vi "Data_folder_Path.vi"(0 "Data Type":string, 1 "FlushHierarchy":bool, 4 "Short_Name":string, 5 "seconds":dbl) -> (6 "Data Folder":path)   [LabVIEW 2015]
uses:
  Globals/Constants_global.vi
  Globals/Preference_global.vi
panel:
  out "Hierarchy":string[](array[string])
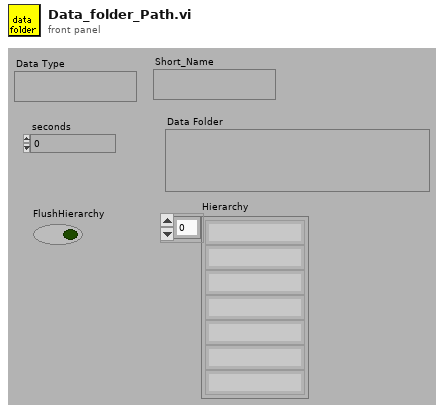
[diagram p1: front panel]
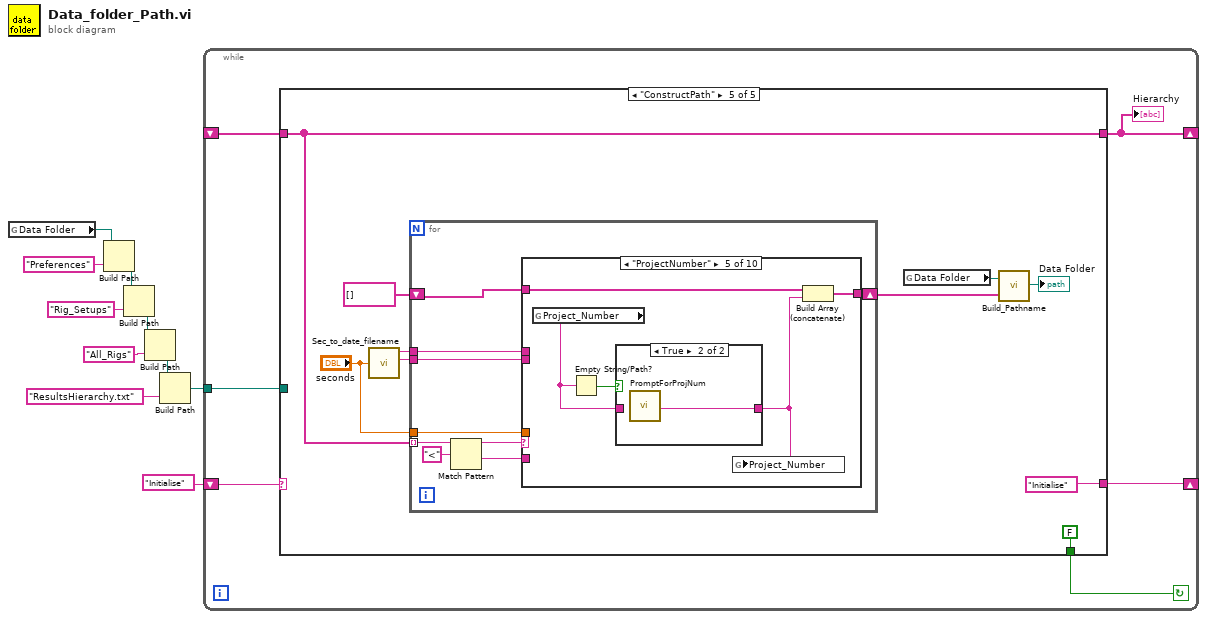
[diagram p0: block diagram]
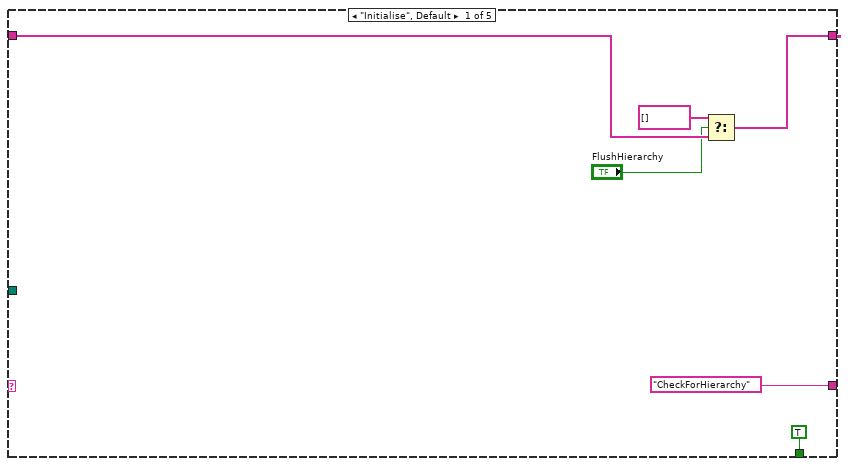
[diagram p2: hidden frame]
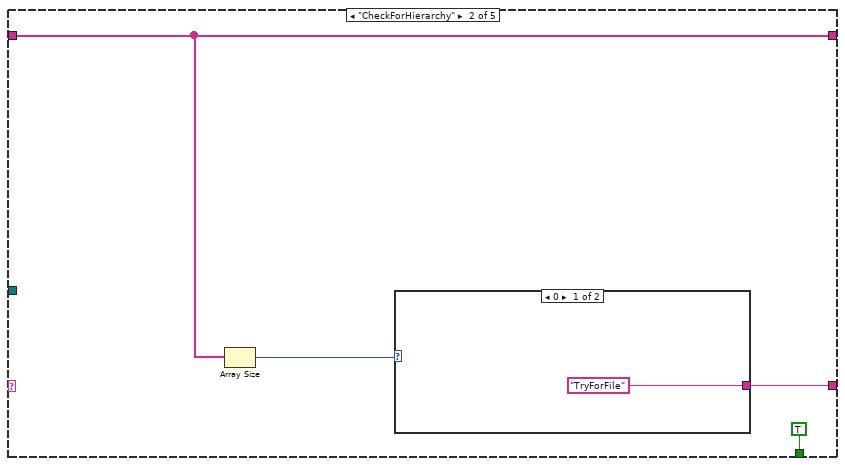
[diagram p3: hidden frame]
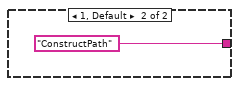
[diagram p4: hidden frame]
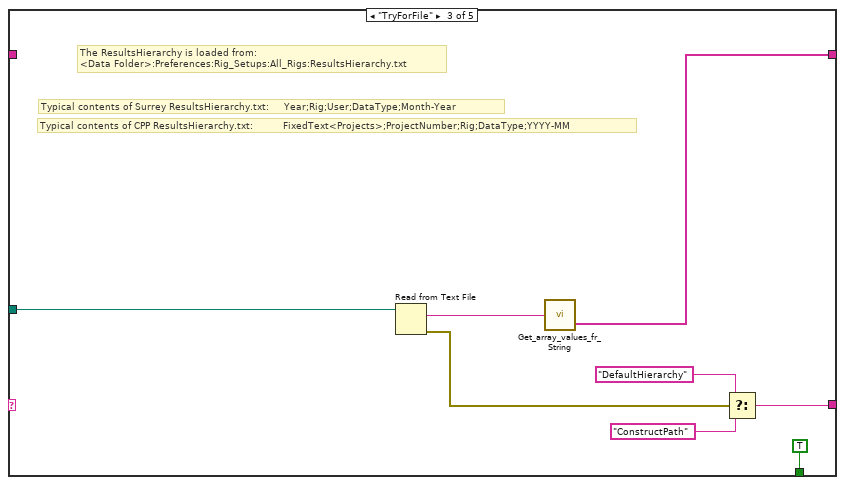
[diagram p5: hidden frame]
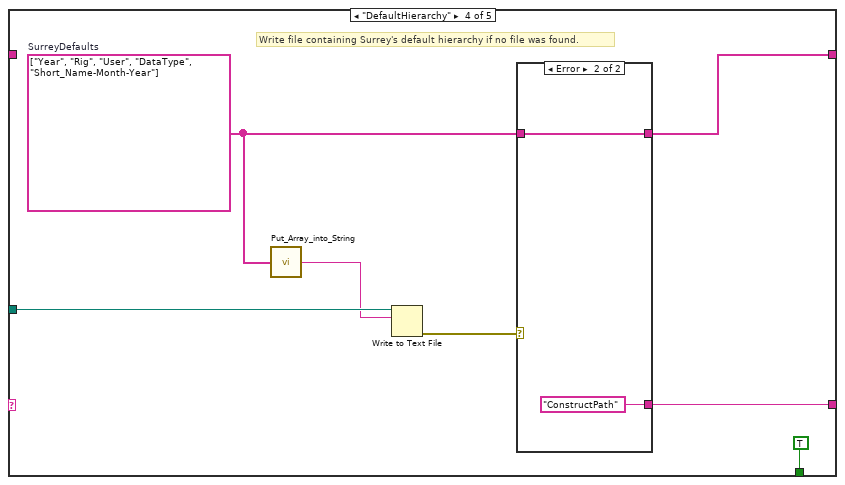
[diagram p6: hidden frame]
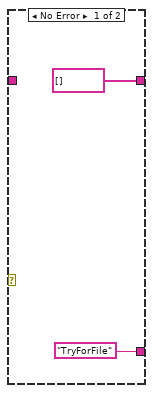
[diagram p7: hidden frame]
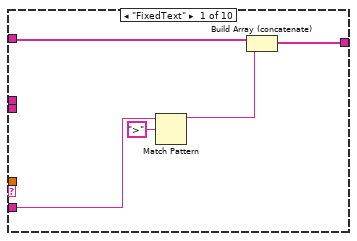
[diagram p8: hidden frame]
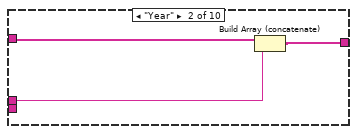
[diagram p9: hidden frame]
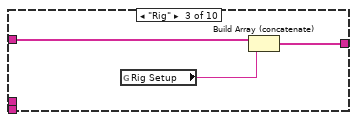
[diagram p10: hidden frame]
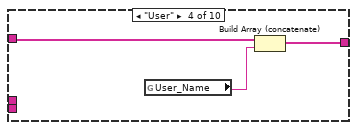
[diagram p11: hidden frame]
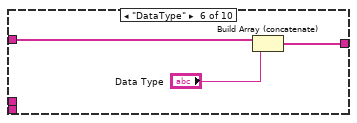
[diagram p13: hidden frame]
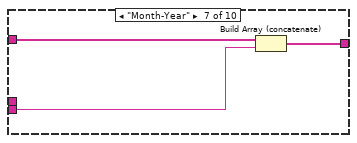
[diagram p14: hidden frame]
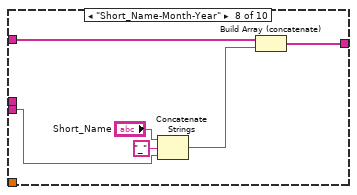
[diagram p15: hidden frame]
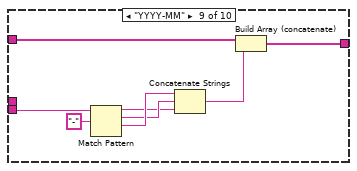
[diagram p16: hidden frame]
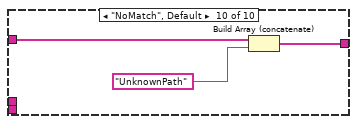
[diagram p17: hidden frame]
diagram:
  n1 = global read "Constants_global.vi" "Data Folder"() -> (w7:path)
  n2 = Build Path(base path=w7, name or relative path="Preferences") -> (appended path=w8:path)
  n3 = Build Path(base path=w8, name or relative path="Rig_Setups") -> (appended path=w1:path)
  n4 = Build Path(base path=w1, name or relative path="All_Rigs") -> (appended path=w5:path)
  n5 = Build Path(base path=w5, name or relative path="ResultsHierarchy.txt") -> (appended path=w2:path)
  n6 = while {
    shift-right: [w14] -> _
    shift-left: _ -> [w15]
    shift-right: [w13] -> _
    shift-left: "Initialise" ("t") -> [w16]
    tunnel: w2 -> [w11]
    stop <- w12 continue-if-true
    n7 = case shown="\"ConstructPath\"" w16 {
      tunnel: w15 -> [w22 w24 _ _ w50]
      tunnel: [w21 w24 w36 w39 w50] -> w14
      tunnel: ["CheckForHierarchy" ("t") w25 w35 w37 "Initialise" ("t")] -> w13
      tunnel: [TRUE TRUE TRUE TRUE FALSE] -> w12
      tunnel: w11 -> [_ _ w29 w42 _]
      frame "Initialise", Default {
        n8 = Select(t=string[] [], s="FlushHierarchy", f=w22) -> (s? t:f=w21:string[])
      }
      frame "CheckForHierarchy" {
        n9 = Array Size(array=w24) -> (size(s)=w26:i32)
        n10 = case shown="0" w26 {
          tunnel: ["TryForFile" ("t") "ConstructPath" ("t")] -> w25
          frame 0 {
          }
          frame 1, Default {
          }
        }
      }
      frame "TryForFile" {
        # "The ResultsHierarchy is loaded from:\n<Data Folder>:Preferences:Rig_Setups:All_Rigs:ResultsHierarchy.txt"
        # "Typical contents of CPP ResultsHierarchy.txt:          FixedText<Projects>;ProjectNumber;Rig;DataType;YYYY-MM"
        # "Typical contents of Surrey ResultsHierarchy.txt:     Year;Rig;User;DataType;Month-Year"
        n11 = Read from Text File(file (use dialog)=w29) -> (text=w31:string, error out=w30:errorcluster)  [unwired: 3 in, 2 out]
        n12 = call "Get_array_values_fr_String.vi"("String Value"=w31) -> ("String array"=w36:string[])  [unwired: 1 out]
        n13 = Select(t="DefaultHierarchy", s=w30, f="ConstructPath" ("t")) -> (s? t:f=w35:string)
      }
      frame "DefaultHierarchy" {
        w38 = string[] ["Year", "Rig", "User", "DataType", "Short_Name-Month-Year"]  # SurreyDefaults
        # "Write file containing Surrey's default hierarchy if no file was found."
        n14 = call "Put_Array_into_String.vi"("String array"=w38) -> ("String Value"=w41:string)
        n15 = Write to Text File(file (use dialog)=w42, text=w41) -> (error out=w40:errorcluster)  [unwired: 2 in, 2 out]
        n16 = case shown="Error" w40 {
          tunnel: [string[] [] ("SurreyDefaults") w47] -> w39
          tunnel: w38 -> [_ w47]
          tunnel: ["TryForFile" ("t") "ConstructPath" ("t")] -> w37
          frame No Error {
          }
          frame Error {
          }
        }
      }
      frame "ConstructPath" {
        n17 = call "Sec_to_date_filename.vi"("seconds"="seconds") -> ("Year"=w55:string, "Month"=w54:string)  [unwired: 2 out]
        n18 = for {
          shift-right: [w66] -> w53
          shift-left: string[] [] -> [w65]
          tunnel: w50 -> [w61] mode=indexing
          tunnel: w54 -> [w64]
          tunnel: w55 -> [w63]
          tunnel: "seconds" -> [w62]
          n19 = Match Pattern(string=w61, regular expression="<") -> (before substring=w60:string, after substring=w58:string)  [unwired: 1 in, 2 out]
          n20 = case shown="\"ProjectNumber\"" w60 {
            tunnel: [w71 w74 w76 w80 w85 w90 w93 w99 w105 w110] -> w66
            tunnel: w65 -> [w70 w73 w75 w78 w84 w89 w92 w98 w104 w109]
            tunnel: w64 -> [_ _ _ _ _ _ w91 w95 w107 _]
            tunnel: w63 -> [_ w72 _ _ _ _ _ _ _ _]
            tunnel: w62 -> [_ _ _ _ _ _ _ _ _ _]
            tunnel: w58 -> [w69 _ _ _ _ _ _ _ _ _]
            frame "FixedText" {
              n21 = Match Pattern(string=w69, regular expression=">") -> (before substring=w67:string)  [unwired: 1 in, 3 out]
              n22 = Build Array (concatenate)(w70, w67) -> (w71:string[])
            }
            frame "Year" {
              n23 = Build Array (concatenate)(w73, w72) -> (w74:string[])
            }
            frame "Rig" {
              n24 = global read "Preference_global.vi" "Rig Setup"() -> (w77:string)
              n25 = Build Array (concatenate)(w75, w77) -> (w76:string[])
            }
            frame "User" {
              n26 = global read "Preference_global.vi" "User_Name"() -> (w79:string)
              n27 = Build Array (concatenate)(w78, w79) -> (w80:string[])
            }
            frame "ProjectNumber" {
              n28 = global read "Preference_global.vi" "Project_Number"() -> (w81:string)
              n29 = Empty String/Path?(string/path=w81) -> (empty?=w83:bool)
              n30 = case shown="True" w83 {
                tunnel: [w86 w87] -> w82
                tunnel: w81 -> [w86 _]
                frame False {
                }
                frame True {
                  n31 = call "PromptForProjNum.vi"() -> ("ProjectNumber"=w87:string)  [unwired: 17 in, 2 out]
                }
              }
              n32 = global write "Preference_global.vi" "Project_Number"(w82) -> ()
              n33 = Build Array (concatenate)(w84, w82) -> (w85:string[])
            }
            frame "DataType" {
              n34 = Build Array (concatenate)(w89, "Data Type") -> (w90:string[])
            }
            frame "Month-Year" {
              n35 = Build Array (concatenate)(w92, w91) -> (w93:string[])
            }
            frame "Short_Name-Month-Year" {
              n36 = Concatenate Strings("Short_Name", "_" ("string"), w95) -> (w94:string)
              n37 = Build Array (concatenate)(w98, w94) -> (w99:string[])
            }
            frame "YYYY-MM" {
              n38 = Match Pattern(string=w107, regular expression="-") -> (before substring=w101:string, match substring=w102:string, after substring=w103:string)  [unwired: 1 in, 1 out]
              n39 = Concatenate Strings(w103, w102, w101) -> (w100:string)
              n40 = Build Array (concatenate)(w104, w100) -> (w105:string[])
            }
            frame "NoMatch", Default {
              n41 = Build Array (concatenate)(w109, "UnknownPath" ("element")) -> (w110:string[])
            }
          }
        }
        n42 = global read "Constants_global.vi" "Data Folder"() -> (w51:path)
        n43 = call "Build_Pathname.vi"("PathElements"=w53, "PathnameIn"=w51) -> ("AppendedPath"=→"Data Folder":path)
      }
    }
    "Hierarchy" <- w14
  }
